vi "ConsumeSign.vi"(8 "error in (no error)":errorcluster, 11 "PathTokenizer in":refnum<class "PathTokenizer.lvclass">) -> (0 "error out":errorcluster, 3 "PathTokenizer out":refnum<class "PathTokenizer.lvclass">)   [LabVIEW 2019, in "PathTokenizer.lvclass"]
uses:
  PathTokenizer.lvclass
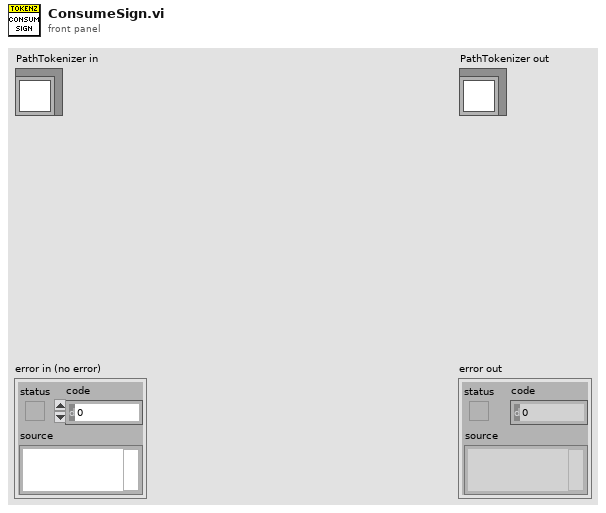
[diagram p1: front panel]
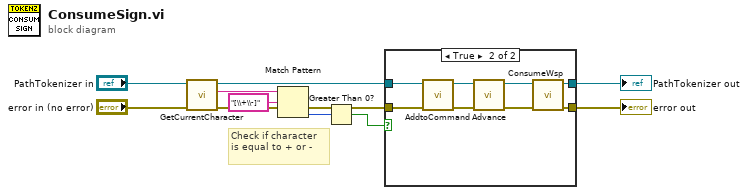
[diagram p0: block diagram]
diagram:
  # "Check if character is equal to + or -"
  n1 = call "GetCurrentCharacter.vi"("error in (no error)"="error in (no error)", "PathTokenizer in"="PathTokenizer in") -> ("error out"=w2:errorcluster, "Current Character"=w8:string, "PathTokenizer out"=w5:refnum<class "PathTokenizer.lvclass">)  [unwired: 7 in]
  n2 = Match Pattern(string=w8, regular expression="[\\+\\-]") -> (offset past match=w6:i32)  [unwired: 1 in, 3 out]
  n3 = Greater Than 0?(x=w6) -> (x > 0?=w3:bool)
  n4 = case shown="True" w3 {
    tunnel: w5 -> [w12 w15]
    tunnel: [w12 w19] -> w4
    tunnel: [w11 w17] -> w1
    tunnel: w2 -> [w11 w13]
    frame False {
    }
    frame True {
      n5 = call "AddtoCommand.vi"("error in (no error)"=w13, "PathTokenizer in"=w15) -> ("error out"=w14:errorcluster, "PathTokenizer out"=w16:refnum<class "PathTokenizer.lvclass">)  [unwired: 8 in]
      n6 = call "Advance.vi"("error in (no error)"=w14, "PathTokenizer in"=w16) -> ("error out"=w18:errorcluster, "PathTokenizer out"=w20:refnum<class "PathTokenizer.lvclass">)  [unwired: 8 in]
      n7 = call "ConsumeWsp.vi"("error in (no error)"=w18, "PathTokenizer in"=w20) -> ("error out"=w17:errorcluster, "PathTokenizer out"=w19:refnum<class "PathTokenizer.lvclass">)  [unwired: 8 in]
    }
  }
  "error out" <- w1
  "PathTokenizer out" <- w4
